vi "Write Controller Data.vi"(10 "Controller Data":T1 {"Force Error" format="%.1f"; "Force Demand" format="%.1f"}, 11 "Logger in":refnum<class "LoggerDatalog.lvclass">) -> (3 "Logger out":refnum<class "LoggerDatalog.lvclass">)   [LabVIEW 2013, in "LoggerDatalog.lvclass"]
uses:
  LoggerDatalog.lvclass
  Typedefs/ControllerData.ctl
  Typedefs/ForceDemand.ctl
  LoggerDatalog.lvclass/LoggerDatalog.ctl
  Typedefs/M2AADTTypedefs.lvlib
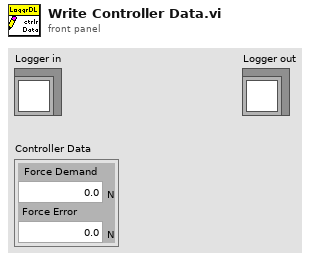
[diagram p1: front panel]
types:
  T1 = typedef "M2AADTTypedefs.lvlib/ControllerData.ctl" = cluster{"Force Demand":T2, "Force Error":T2}
  T2 = typedef "M2AADTTypedefs.lvlib/ForceDemand.ctl" = dbl[unit]
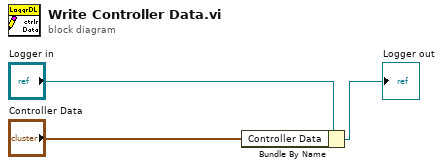
[diagram p0: block diagram]
diagram:
  n1 = Bundle By Name(cluster="Logger in", "Controller Data"="Controller Data") -> (→"Logger out":refnum<class "LoggerDatalog.lvclass">)
